vi "Pre Launch Init.vi"(11 "ServiceManager-Comms in":refnum<class "ServiceManager-Comms.lvclass">) -> (0 "error out":errorcluster, 3 "ServiceManager-Comms out":refnum<class "ServiceManager-Comms.lvclass">)   [LabVIEW 2020, in "ServiceManager.lvlib" / "ServiceManager-Comms.lvclass"]
doc: "(<B>Filename</B>: Actor Framework.lvlib:Actor.lvclass:Pre Launch Init.vi)\n\nDefines behavior that occurs after the Launch Nested Actor method is invoked but before the actor's Actor Core method begins running.\n\nBy default, this method does nothing. A descendant class may override it to define behavior."
uses:
  ServiceManager-Comms.lvclass
  <vilib>/ActorFramework/Actor/Actor.lvclass
  ServiceManager-Comms Messages/WaitForConnect Msg/WaitForConnect Msg.lvclass
  C:/Program Files (x86)/National Instruments/LabVIEW 2020/vi.lib/ActorFramework/Actor/Actor.lvclass
  C:/Users/taylo/Projects/g-go-service-fwrk/scratchpad/ServiceManagerBeta/ServiceManager/ServiceManager-Comms/ServiceManager-Comms.lvclass
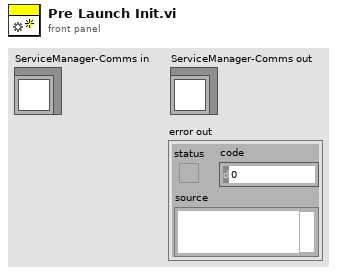
[diagram p1: front panel]
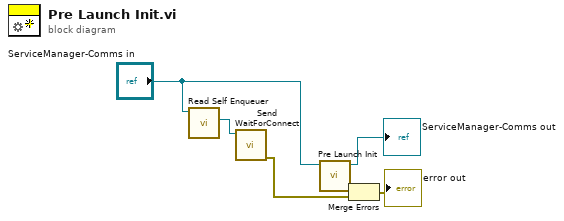
[diagram p0: block diagram]
diagram:
  n1 = call <vilib>:"Read Self Enqueuer.vi"("Actor"="ServiceManager-Comms in") -> ("Self Enqueuer"=w3:refnum<class "Message Enqueuer.lvclass">)  [unwired: 10 in]
  n2 = call "Send WaitForConnect.vi"("Message Enqueuer"=w3) -> ("error out"=w1:errorcluster)  [unwired: 9 in, 1 out]
  n3 = call-parent "Pre Launch Init.vi"("Actor in"="ServiceManager-Comms in") -> ("error out"=w6:errorcluster, "Actor out"=→"ServiceManager-Comms out":refnum<class "ServiceManager-Comms.lvclass">)  [unwired: 9 in]
  n4 = Merge Errors(w6, w1) -> (→"error out":errorcluster)
